vi "Vision Global Data.vi"() -> ()   [LabVIEW 2012]
uses:
  TargetData.ctl
panel:
  in  "Location":T1
  out "targetGot":bool
  in  "getTarget":bool=TRUE
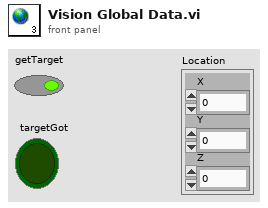
[diagram p1: front panel]
types:
  T1 = typedef "TargetData.ctl" = cluster{"X":dbl, "Y":dbl, "Z":dbl}
diagram:
